vi "PTO Operation.vi"(0 "Left Motor Power In":dbl, 1 "PTO  Engaged IN?":bool, 2 "Right Motor Power In":dbl) -> (7 "Left Motor Power Out":dbl, 8 "PTO Engaged? Out":bool, 9 "Right Motor Power Out":dbl)   [LabVIEW 2016]
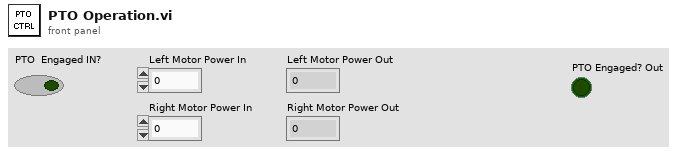
[diagram p1: front panel]
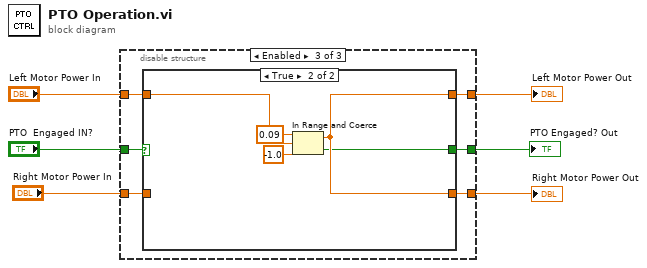
[diagram p0: block diagram]
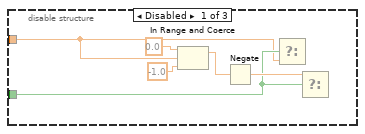
[diagram p2: hidden frame]
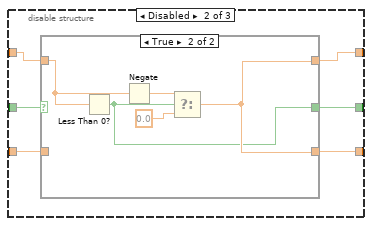
[diagram p3: hidden frame]
diagram:
  n1 = disable-structure shown="Enabled" {
    disable-tunnel: "PTO  Engaged IN?" -> [w8 w18 w32]
    disable-tunnel: "Left Motor Power In" -> [w7 w17 w31]
    disable-tunnel: "Right Motor Power In" -> [_ w16 w29]
    disable-tunnel: [_ w15 w30] -> w3
    disable-tunnel: [_ w14 w28] -> w2
    disable-tunnel: [_ w13 w27] -> w1
    frame Disabled {
      n2 = In Range and Coerce(upper limit=0.0, x=w7, lower limit=-1.0) -> (coerced(x)=w10:dbl)  [unwired: 1 out]
      n3 = Negate(x=w10) -> (-x=w9:dbl)
      n4 = Select(s=w8, f=w7) -> ()  [unwired: 1 in, 1 out]
      n5 = Select(t=w9, s=w8) -> ()  [unwired: 1 in, 1 out]
    }
    frame Disabled {
      n6 = case shown="True" w18 {
        selector: w18 -> [w19 _]
        tunnel: w17 -> [w21 w26]
        tunnel: w16 -> [w20 _]
        tunnel: [w21 w24] -> w15
        tunnel: [w20 w24] -> w14
        tunnel: [w19 w23] -> w13
        frame False {
        }
        frame True {
          n7 = Less Than 0?(x=w26) -> (x < 0?=w23:bool)
          n8 = Negate(x=w26) -> (-x=w22:dbl)
          n9 = Select(t=w22, s=w23, f=0.0 ("t")) -> (s? t:f=w24:dbl)
        }
      }
    }
    frame Enabled {
      n10 = case shown="True" w32 {
        selector: w32 -> [w33 _]
        tunnel: w31 -> [w35 w40]
        tunnel: [w35 w39] -> w30
        tunnel: w29 -> [w34 _]
        tunnel: [w34 w39] -> w28
        tunnel: [w33 w36] -> w27
        frame False {
        }
        frame True {
          n11 = In Range and Coerce(upper limit=0.09, x=w40, lower limit=-1.0) -> (coerced(x)=w39:dbl, In Range?=w36:bool)
        }
      }
    }
  }
  "PTO Engaged? Out" <- w1
  "Right Motor Power Out" <- w2
  "Left Motor Power Out" <- w3
